vi "Teleop.vi"(10 "Match Info":T1={"Autonomous Elapsed Seconds"=0.0, "TeleOp Elapsed Seconds"=0.0, "Disabled Elapsed Seconds"=0.0, "Visited Autonomous"=FALSE, "Visited TeleOp"=FALSE, "Visited Disabled"=FALSE, "Autonomous Settings"={"Autonomous Style"=enum."Independent", "VI Refnum"=refnum}}, 11 "Call Context":T2) -> ()   [LabVIEW 2016]
doc: "This VI is called for each TeleOp packet received from the DS where the robot is not disabled. It is often used to read from the joysticks and update I/O or to update setpoints for timed control loops. It should complete and return within 20 milliseconds or it may miss DS packets."
uses:
  <vilib>/Rock Robotics/WPI/DriverStation/WPI_DriverStationDerivedRobotMode.ctl
  <vilib>/Rock Robotics/WPI/DriverStation/WPI_DriverStationMatch Info.ctl
  <vilib>/Rock Robotics/WPI/ThirdParty/CanMotor/TalonSRX/WPI_CANTalonSRX_APIFeedbackSelect.ctl
  <vilib>/Rock Robotics/WPI/ThirdParty/CanMotor/TalonSRX/WPI_CANTalonSRX_APIControlMode.ctl
  <vilib>/Rock Robotics/WPI/Utilities/WPI_GetSetVariantRefNum.vi
  <vilib>/Rock Robotics/Network Tables/NT Write Boolean Array.vi
  <vilib>/Rock Robotics/Network Tables/NT Write Numeric Array.vi
  <vilib>/Rock Robotics/Network Tables/NT Read Boolean.vi
  <vilib>/Rock Robotics/Network Tables/NT Read Number.vi
  Robot Global Data.vi
  <vilib>/Rock Robotics/Network Tables/NT Write Boolean.vi
panel:
  out "Battery Voltage":dbl
  out "Current":dbl
  out "SensorPosRotations":dbl
  out "Motor output Plot":cluster{"Applied Throttle":dbl}(graph)
  out "Target RPM":dbl
  out "SensorRPM Velocity RPM":dbl
  out "Applied Output":dbl
  out "Speed Closed Loop Plots":cluster{dbl, "Sensor Velocity":dbl}(graph)
  in  "Enable":bool=TRUE
  in  "Reset":bool
  out "Table":string[][](table)
  out "Encoder Velocity":dbl
  out "Sample Slider 0":dbl(slide) scale=0.0..5.0
  out "Sample Boolean 1":bool
  out "Sample Boolean 0":bool
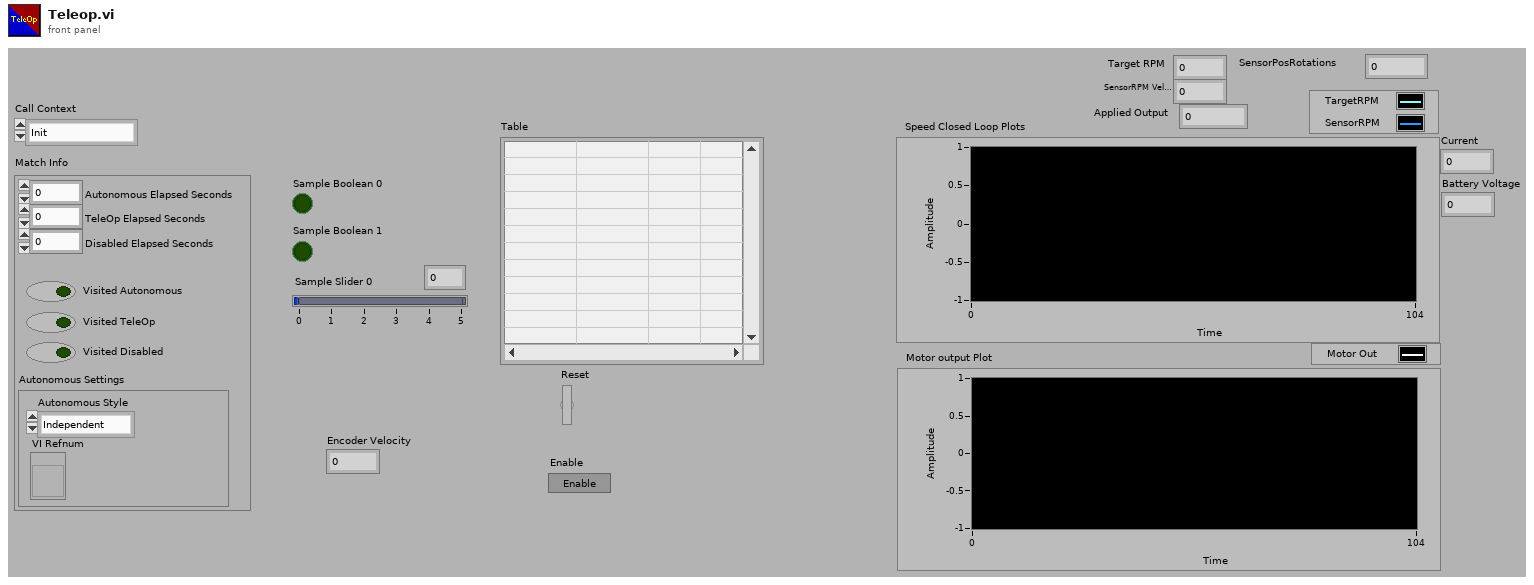
[diagram p1: front panel]
types:
  T1 = typedef "WPI_DriverStationMatch Info.ctl" = cluster{"Autonomous Elapsed Seconds":dbl, "TeleOp Elapsed Seconds":dbl, "Disabled Elapsed Seconds":dbl, "Visited Autonomous":bool, "Visited TeleOp":bool, "Visited Disabled":bool, "Autonomous Settings":cluster{"Autonomous Style":enum16{"Iterative", "Independent"}, "VI Refnum":refnum<vi>}}
  T2 = typedef "WPI_DriverStationDerivedRobotMode.ctl" = enum16{"Init", "Execute", "Stop"}
  T3 = typedef "WPI_CANTalonSRX_APIFeedbackSelect.ctl" = enum16{"Digital Quadrature Encoder", "Analog Potentiometer", "Analog Encoder", "Count on Quad-A (Rising-Edge)", "Count on Quad-A (Falling-Edge)", "CTR Magnetic Enc (Absolute)", "CTR Magnetic Enc (Relative)", "Pulse Width"}
  T4 = typedef "WPI_JoystickDevRef.ctl" = cluster{"Device":T5}
  T5 = typedef "WPI_JoystickDeviceEnum.ctl" = enum16{"USB 0", "USB 1", "USB 2", "USB 3", "USB 4", "USB 5"}
  T6 = typedef "WPI_RobotDriveDevRef.ctl" = cluster{"DevStatus":errorcluster, "Motors[]":T7[], "Square Inputs":bool, "Max Output":dbl}
  T7 = typedef "WPI_MotorControlDeviceRef.ctl" = cluster{"DeviceStatus":errorcluster, "Type":T8, "PWM":cluster{"PWM Channel":T9, "DeadBand":T10}, "CAN":cluster{"Device Number":u8, "SetOutput VI Ref":variant, "GetOutput VI Ref":variant, "Enable VI Ref":variant, "Disable VI Ref":variant, "Data":variant}, "Invert":bool}
  T8 = typedef "WPI_MotorControlType.ctl" = enum16{"PWM", "CAN"}
  T9 = typedef "FPGA_DIOPWMChannel.ctl" = enum8{"PWM 0", "PWM 1", "PWM 2", "PWM 3", "PWM 4", "PWM 5", "PWM 6", "PWM 7", "PWM 8", "PWM 9", "PWM MXP 0", "PWM MXP 1", "PWM MXP 2", "PWM MXP 3", "PWM MXP 4", "PWM MXP 5", "PWM MXP 6", "PWM MXP 7", "PWM MXP 8", "PWM MXP 9", "Invalid"}
  T10 = typedef "WPI_PWMDeadband.ctl" = cluster{"Name":string, "maxPositivePwm":i32, "minPositivePwm":i32, "centerPwm":i32, "maxNegativePwm":i32, "minNegativePwm":i32, "angularRange":u16}
  T11 = typedef "WPI_CANTalonSRX_GlobalStatus.ctl" = cluster{"Applied Throttle":dbl, "Module Enabled":bool, "CAN Error":errorcluster, "Closed Loop Error":dbl, "Forward Limit Switch Closed":bool, "Reverse Limit Switch Closed":bool, "Sensor Position":dbl, "Sensor Velocity":dbl, "Current":dbl, "Sticky Fault - Over Temp":bool, "Sticky Fault - Under Voltage":bool, "Sticky Fault - Forward Limit":bool, "Sticky Fault - Reverse Limit":bool, "Sticky Fault - Forward Soft Limit":bool, "Sticky Fault - Reverse Soft Limit":bool, "Brake is Enabled":bool, "Encoder Position":dbl, "Encoder Velocity":dbl, "Encoder Index Count":dbl, "Encoder A Pin State":bool, "Encoder B Pin State":bool, "Encoder Index Pin State":bool, "Analog In":dbl, "Analog In Velocity":dbl, "Temperature (C)":dbl, "Battery Voltage":dbl, "Control 5 Is Supported":bool, "Current Profile Slot Select":dbl, "Pos Div 8":bool, "Vel Div 4":bool, "Pulse Width Position":i32, "Pulse Width Velocity":i32, "Pulse Width Rise To Rise (us)":i32, "Pulse Width Rise To Fall (us)":i32, "Mot Prof Active Is Under Run":bool, "Mot Prof Active Has Under Run":bool, "Mot Prof Active Is Last":bool, "Mot Prof Active Velocity Only":bool, "Mot Prof Active Is Valid":bool, "Mot Prof Buffer Is Full":bool, "Mot Prof Active Profile Slot Select":i32, "Mot Prof NextID":i32, "Mot Prof Count":i32, "Mot Prof Active Velocity":dbl, "Mot Prof Active Position":dbl, "Mot Prof Output Enable":i32, "UsageFrame":u32}
  T12 = typedef "WPI_DigitalInputDevRef.ctl" = cluster{"DevStatus":errorcluster, "DIO Channel":T13}
  T13 = typedef "FPGA_DIOChannel.ctl" = enum8{"DIO 0", "DIO 1", "DIO 2", "DIO 3", "DIO 4", "DIO 5", "DIO 6", "DIO 7", "DIO 8", "DIO 9", "DIO MXP 0", "DIO MXP 1", "DIO MXP 2", "DIO MXP 3", "DIO MXP 4", "DIO MXP 5", "DIO MXP 6", "DIO MXP 7", "DIO MXP 8", "DIO MXP 9", "DIO MXP 10", "DIO MXP 11", "DIO MXP 12", "DIO MXP 13", "DIO MXP 14", "DIO MXP 15", "SPI Port CS1", "SPI Port CS2", "SPI Port CS3", "SPI Port MISO", "SPI Port MOSI", "Invalid"}
  T14 = typedef "WPI_CANTalonSRX_APIControlMode.ctl" = enum8{"Percent VBus", "Speed", "Position", "Slave", "Unchanged / Invalid", "Voltage Compensation", "Current", "Motion Profile", "Motion Magic"}
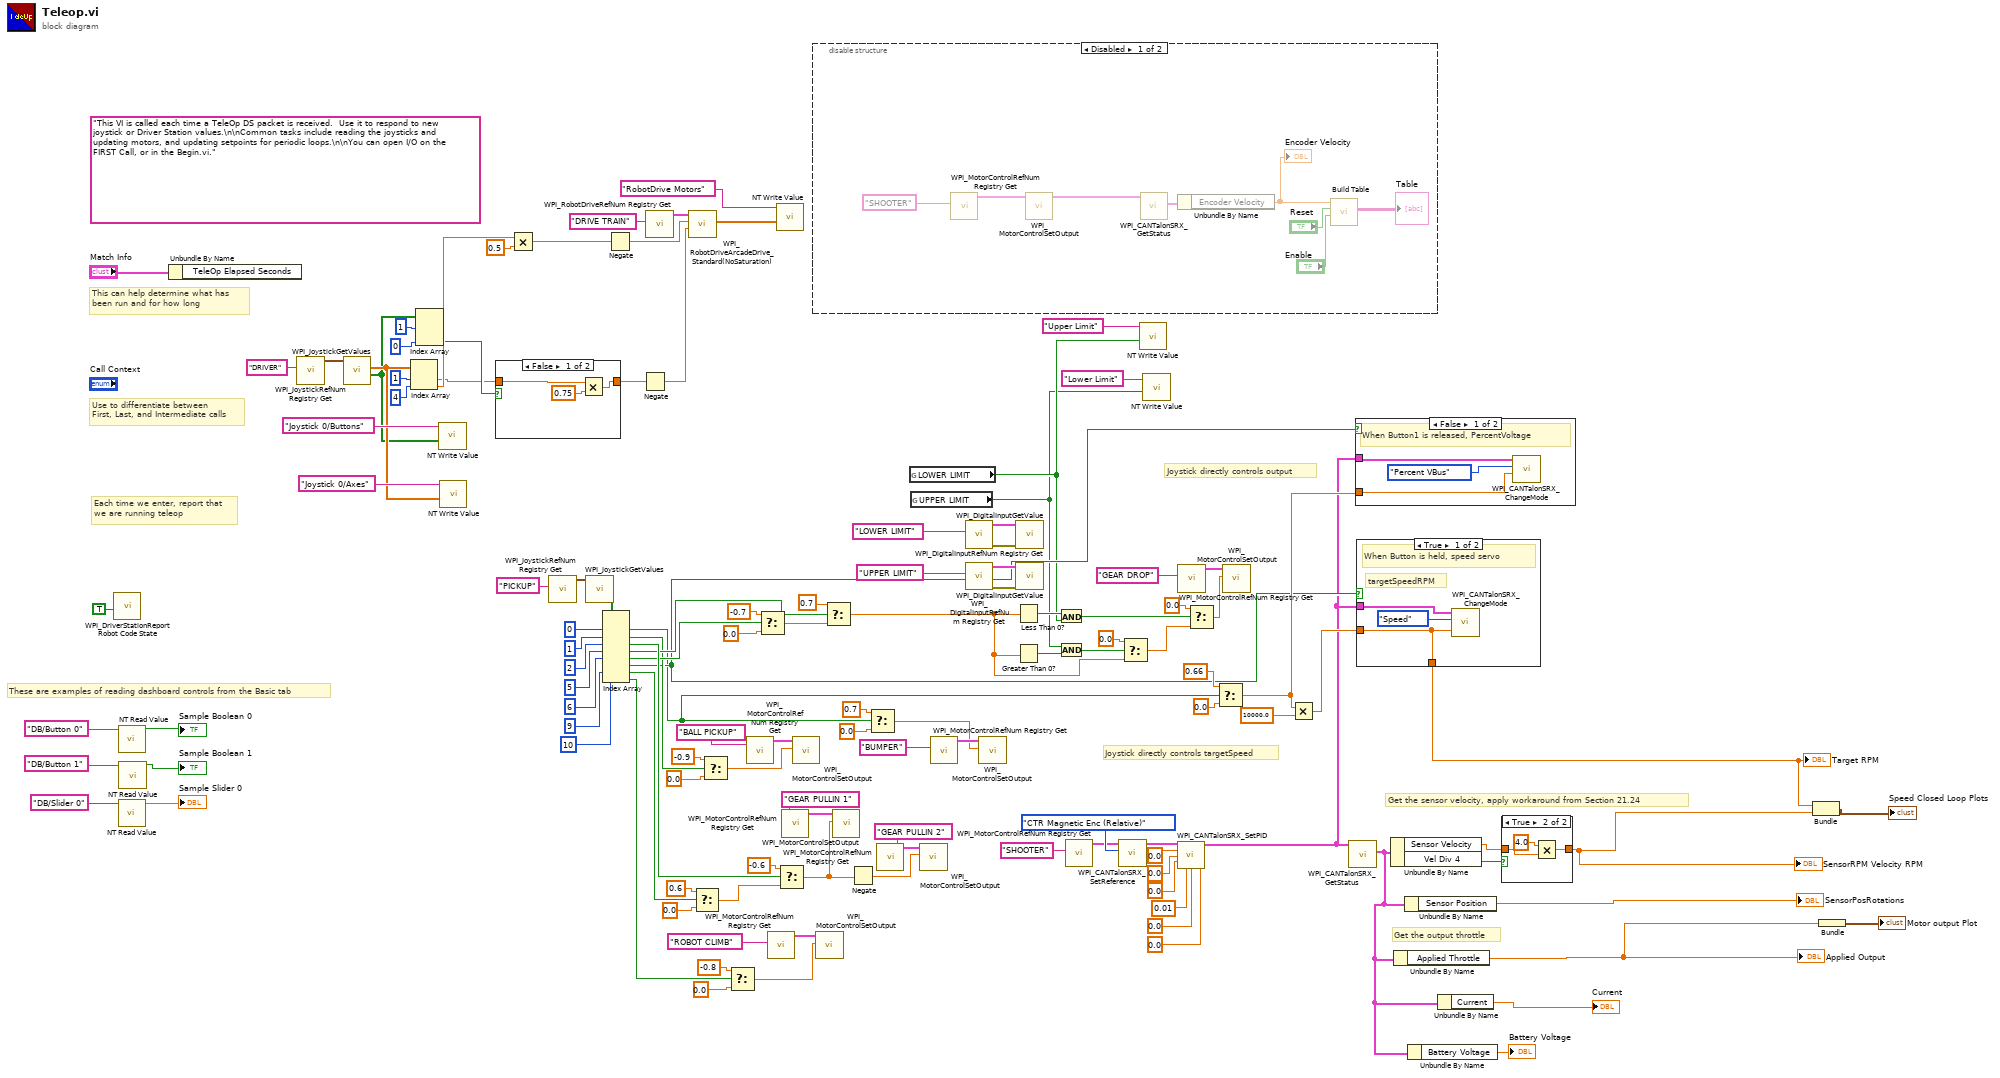
[diagram p0: block diagram]
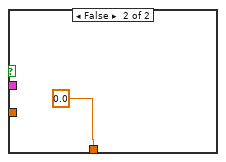
[diagram p6: hidden frame]
diagram:
  (unwired) "This VI is called each time a TeleOp DS packet is received.  Use it to respond to new joystick or Driver Station values.\n\nCommon tasks include reading the joysticks and updating motors, and updating setpoints for periodic loops.\n\nYou can open I/O on the FIRST Call, or in the Begin.vi."
  # "Get the output throttle"
  # "Get the sensor velocity, apply workaround from Section 21.24"
  # "Joystick directly controls targetSpeed"
  # "Joystick directly controls output"
  # "These are examples of reading dashboard controls from the Basic tab"
  # "Each time we enter, report that\nwe are running teleop"
  # "Use to differentiate between\nFirst, Last, and Intermediate calls"
  # "This can help determine what has\nbeen run and for how long"
  n1 = call <vilib>:"WPI_DriverStationReport Robot Code State.vi"("TeleOp"=TRUE ("Autonomous")) -> ()  [unwired: 10 in, 1 out]
  n2 = call-poly <vilib>:"NT Read Value.vi"("Name"="DB/Button 0" ("refnum name")) -> ("Boolean"=→"Sample Boolean 0":bool)  [unwired: 9 in, 1 out]
  n3 = call-poly <vilib>:"NT Read Value.vi"("Name"="DB/Slider 0" ("refnum name")) -> ("Numeric"=→"Sample Slider 0":dbl)  [unwired: 9 in, 1 out]
  n4 = call-poly <vilib>:"NT Read Value.vi"("Name"="DB/Button 1" ("refnum name")) -> ("Boolean"=→"Sample Boolean 1":bool)  [unwired: 9 in, 1 out]
  n5 = Unbundle By Name("Match Info") -> ()  [unwired: 1 out]
  n6 = call <vilib>:"WPI_JoystickRefNum Registry Get.vi"("refnum name"="DRIVER") -> ("JoystickDevRef"=w121:T4)  [unwired: 1 in, 9 out]
  n7 = call <vilib>:"WPI_JoystickGetValues.vi"("JoystickDevRef"=w121) -> ("Buttons"=w79:bool[], "Axes"=w117:dbl[])  [unwired: 6 in, 3 out]
  n8 = Index Array(array=w117, index #1=1 ("index"), index #2=4 ("index")) -> (element #1=w22:dbl, element #2=w75:dbl)
  n9 = Index Array(array=w79, index #1=1 ("index"), index #3=0 ("index")) -> (element #3=w23:bool)  [unwired: 1 in, 2 out]
  n10 = call-poly <vilib>:"NT Write Value.vi"("Boolean Array"=w79, "Name"="Joystick 0/Buttons") -> ()  [unwired: 9 in, 1 out]
  n11 = call-poly <vilib>:"NT Write Value.vi"("Numeric Array"=w117, "Name"="Joystick 0/Axes") -> ()  [unwired: 9 in, 1 out]
  n12 = case shown="False" w23 {
    tunnel: [w127 w129] -> w21
    tunnel: w22 -> [w126 w129]
    frame False {
      n13 = Multiply(x=w126, y=0.75) -> (x*y=w127:dbl)
    }
    frame True {
    }
  }
  n14 = Multiply(x=w75, y=0.5) -> (x*y=w66:dbl)
  n15 = call <vilib>:"WPI_JoystickRefNum Registry Get.vi"("refnum name"="PICKUP") -> ("JoystickDevRef"=w108:T4)  [unwired: 1 in, 9 out]
  n16 = call <vilib>:"WPI_JoystickGetValues.vi"("JoystickDevRef"=w108) -> ("Buttons"=w106:bool[])  [unwired: 6 in, 4 out]
  n17 = Index Array(array=w106, index #1=0 ("index"), index #2=1 ("index"), index #3=2 ("index"), index #4=5 ("index"), index #5=6 ("index"), index #7=9 ("index"), index #8=10 ("index")) -> (element #1=w31:bool, element #2=w82:bool, element #3=w89:bool, element #4=w88:bool, element #5=w87:bool, element #6=w34:bool, element #7=w17:bool, element #8=w5:bool)  [unwired: 1 in]
  n18 = Negate(x=w66) -> (-x=w65:dbl)
  n19 = Negate(x=w21) -> (-x=w67:dbl)
  n20 = call <vilib>:"WPI_RobotDriveRefNum Registry Get.vi"("refnum name"="DRIVE TRAIN") -> ("RobotDriveDevRef"=w123:T6)  [unwired: 1 in, 9 out]
  n21 = call <vilib>:"WPI_RobotDriveArcadeDrive_Standard(NoSaturation).vi"("Y axis value"=w67, "X axis value"=w65, "RobotDriveDevRef"=w123) -> ("Motor Values"=w110:dbl[])  [unwired: 1 in, 7 out]
  n22 = Select(t=0.6, s=w17, f=0.0) -> (s? t:f=w19:dbl)
  n23 = Select(t=-0.9, s=w82, f=0.0) -> (s? t:f=w84:dbl)
  n24 = Select(t=-0.8, s=w5, f=0.0) -> (s? t:f=w8:dbl)
  n25 = call <vilib>:"WPI_MotorControlRefNum Registry Get.vi"("refnum name"="BALL PICKUP") -> ("MotorControlDevRef"=w86:T7)  [unwired: 9 in, 1 out]
  n26 = Select(t=-0.7, s=w87, f=0.0) -> (s? t:f=w63:dbl)
  n27 = call <vilib>:"WPI_MotorControlRefNum Registry Get.vi"("refnum name"="ROBOT CLIMB") -> ("MotorControlDevRef"=w9:T7)  [unwired: 9 in, 1 out]
  n28 = call-poly <vilib>:"NT Write Value.vi"("Numeric Array"=w110, "Name"="RobotDrive Motors") -> ()  [unwired: 9 in, 1 out]
  n29 = Select(t=-0.6, s=w89, f=w19) -> (s? t:f=w99:dbl)
  n30 = call <vilib>:"WPI_MotorControlRefNum Registry Get.vi"("refnum name"="GEAR PULLIN 1") -> ("MotorControlDevRef"=w104:T7)  [unwired: 9 in, 1 out]
  n31 = call <vilib>:"WPI_MotorControlSetOutput.vi"("Output"=w84, "MotorControlDevRef"=w86) -> ()  [unwired: 7 in, 3 out]
  n32 = disable-structure shown="Disabled" {
    frame Disabled {
      n33 = call <vilib>:"WPI_MotorControlRefNum Registry Get.vi"("refnum name"="SHOOTER") -> ("MotorControlDevRef"=w130:T7)  [unwired: 9 in, 1 out]
      n34 = call <vilib>:"WPI_MotorControlSetOutput.vi"("MotorControlDevRef"=w130) -> ("MotorControlDevRef"=w137:T7)  [unwired: 8 in, 2 out]
      n35 = call <vilib>:"WPI_CANTalonSRX_GetStatus.vi"("CAN Talon SRX Ref"=w137) -> ("Talon SRX Status"=w136:T11)  [unwired: 8 in, 2 out]
      n36 = Unbundle By Name(w136) -> ("Encoder Velocity"=w134:dbl)
      "Encoder Velocity" <- w134
      n37 = call "Build Table"("Enable"="Enable", "Reset"="Reset", "Signals"=w134) -> ("Table"=→"Table":string[][])  [unwired: 2 in, 6 out]
    }
    frame Enabled {
    }
  }
  n38 = call <vilib>:"WPI_MotorControlSetOutput.vi"("Output"=w8, "MotorControlDevRef"=w9) -> ()  [unwired: 7 in, 3 out]
  n39 = Select(t=0.7, s=w88, f=w63) -> (s? t:f=w57:dbl)
  n40 = call <vilib>:"WPI_MotorControlSetOutput.vi"("Output"=w99, "MotorControlDevRef"=w104) -> ()  [unwired: 7 in, 3 out]
  n41 = Negate(x=w99) -> (-x=w98:dbl)
  n42 = Select(t=0.7, s=w31, f=0.0) -> (s? t:f=w28:dbl)
  n43 = call <vilib>:"WPI_MotorControlRefNum Registry Get.vi"("refnum name"="GEAR PULLIN 2") -> ("MotorControlDevRef"=w101:T7)  [unwired: 9 in, 1 out]
  n44 = global read "Robot Global Data.vi" "LOWER LIMIT"() -> (w4:bool)
  n45 = global read "Robot Global Data.vi" "UPPER LIMIT"() -> (w3:bool)
  n46 = call <vilib>:"WPI_MotorControlSetOutput.vi"("Output"=w98, "MotorControlDevRef"=w101) -> ()  [unwired: 7 in, 3 out]
  n47 = call <vilib>:"WPI_MotorControlRefNum Registry Get.vi"("refnum name"="BUMPER") -> ("MotorControlDevRef"=w33:T7)  [unwired: 9 in, 1 out]
  n48 = call <vilib>:"WPI_DigitalInputRefNum Registry Get.vi"("refnum name"="LOWER LIMIT") -> ("error out"=w70:errorcluster, "DigitalInputDevRef"=w71:T12)  [unwired: 9 in]
  n49 = call <vilib>:"WPI_DigitalInputRefNum Registry Get.vi"("refnum name"="UPPER LIMIT") -> ("error out"=w73:errorcluster, "DigitalInputDevRef"=w72:T12)  [unwired: 9 in]
  n50 = call <vilib>:"WPI_MotorControlSetOutput.vi"("Output"=w28, "MotorControlDevRef"=w33) -> ()  [unwired: 7 in, 3 out]
  n51 = Less Than 0?(x=w57) -> (x < 0?=w59:bool)
  n52 = Greater Than 0?(x=w57) -> (x > 0?=w60:bool)
  n53 = call <vilib>:"WPI_DigitalInputGetValue.vi"("error in (no error)"=w70, "DigitalInputDevRef"=w71) -> ()  [unwired: 7 in, 3 out]
  n54 = call <vilib>:"WPI_DigitalInputGetValue.vi"("error in (no error)"=w73, "DigitalInputDevRef"=w72) -> ()  [unwired: 7 in, 3 out]
  n55 = And(x=w59, y=w4) -> (x .and. y?=w61:bool)
  n56 = And(x=w3, y=w60) -> (x .and. y?=w62:bool)
  n57 = call <vilib>:"WPI_MotorControlRefNum Registry Get.vi"("refnum name"="SHOOTER") -> ("MotorControlDevRef"=w45:T7)  [unwired: 9 in, 1 out]
  n58 = call <vilib>:"WPI_CANTalonSRX_SetReference.vi"("Feedback Reference"=WPI_CANTalonSRX_APIFeedbackSelect."CTR Magnetic Enc (Relative)", "CAN Talon SRX Ref"=w45) -> ("CAN Talon SRX Ref"=w44:T7)  [unwired: 8 in, 1 out]
  n59 = Select(t=0.0, s=w62, f=w57) -> (s? t:f=w55:dbl)
  n60 = call-poly <vilib>:"NT Write Value.vi"("Boolean"=w4, "Name"="Upper Limit") -> ()  [unwired: 9 in, 1 out]
  n61 = call-poly <vilib>:"NT Write Value.vi"("Boolean"=w3, "Name"="Lower Limit") -> ()  [unwired: 9 in, 1 out]
  n62 = call <vilib>:"WPI_CANTalonSRX_SetPID.vi"("CAN Talon SRX Ref"=w44, "P"=0.0, "I"=0.0, "D"=0.0, "F"=0.01, "I Zone"=0.0, "Ramp Rate"=0.0) -> ("CAN Talon SRX Ref"=w15:T7)  [unwired: 7 in, 1 out]
  n63 = call <vilib>:"WPI_MotorControlRefNum Registry Get.vi"("refnum name"="GEAR DROP") -> ("MotorControlDevRef"=w96:T7)  [unwired: 9 in, 1 out]
  n64 = Select(t=0.0, s=w61, f=w55) -> (s? t:f=w64:dbl)
  n65 = Select(t=0.66 ("Output"), s=w31, f=0.0) -> (s? t:f=w36:dbl)
  n66 = call <vilib>:"WPI_MotorControlSetOutput.vi"("Output"=w64, "MotorControlDevRef"=w96) -> ()  [unwired: 7 in, 3 out]
  n67 = Multiply(x=w36, y=10000.0) -> (x*y=w39:dbl)
  n68 = call <vilib>:"WPI_CANTalonSRX_GetStatus.vi"("CAN Talon SRX Ref"=w15) -> ("Talon SRX Status"=w26:T11)  [unwired: 8 in, 2 out]
  n69 = case shown="False" w34 {
    tunnel: w15 -> [w139 _]
    tunnel: w36 -> [w138 _]
    frame False {
      # "When Button1 is released, PercentVoltage"
      n70 = call <vilib>:"WPI_CANTalonSRX_ChangeMode.vi"("Output"=w138, "Control Mode"=WPI_CANTalonSRX_APIControlMode."Percent VBus", "CAN Talon SRX Ref"=w139) -> ()  [unwired: 7 in, 2 out]
    }
    frame True {
    }
  }
  n71 = case shown="True" w34 {
    tunnel: w39 -> [w141 _]
    tunnel: w15 -> [w142 _]
    tunnel: [w141 0.0 ("x")] -> w38
    frame True {
      # "targetSpeedRPM"
      # "When Button is held, speed servo"
      n72 = call <vilib>:"WPI_CANTalonSRX_ChangeMode.vi"("Output"=w141, "Control Mode"=WPI_CANTalonSRX_APIControlMode."Speed", "CAN Talon SRX Ref"=w142) -> ()  [unwired: 7 in, 2 out]
    }
    frame False {
    }
  }
  "Target RPM" <- w38
  n73 = Unbundle By Name(w26) -> ("Sensor Velocity"=w48:dbl, "Vel Div 4"=w47:bool)
  n74 = Unbundle By Name(w26) -> ("Applied Throttle"=w40:dbl)
  "Applied Output" <- w40
  n75 = Unbundle By Name(w26) -> ("Sensor Position"=→"SensorPosRotations":dbl)
  n76 = Unbundle By Name(w26) -> ("Battery Voltage"=→"Battery Voltage":dbl)
  n77 = Unbundle By Name(w26) -> ("Current"=→"Current":dbl)
  n78 = case shown="True" w47 {
    tunnel: [w145 w147] -> w46
    tunnel: w48 -> [w145 w146]
    frame False {
    }
    frame True {
      n79 = Multiply(x=4.0, y=w146) -> (x*y=w147:dbl)
    }
  }
  "SensorRPM Velocity RPM" <- w46
  n80 = Bundle("x"=w38, "Sensor Velocity"=w46) -> (→"Speed Closed Loop Plots":cluster{"x":dbl, "Sensor Velocity":dbl})  [unwired: 1 in]
  n81 = Bundle("Applied Throttle"=w40) -> (→"Motor output Plot":cluster{"Applied Throttle":dbl})  [unwired: 1 in]
